vi "Remote Systems Demo.vi"() -> ()   [LabVIEW 2020]
uses:
  Dynamic Combobox/Dynamic Combobox/Options.ctl
  Remote Systems.lvclass
  C:/dev/NI/Dynamic Combobox/Dynamic Combobox/Dynamic Values/Dynamic Values.lvclass
  Dynamic Combobox/Dynamic Combobox/Dynamic Combobox.lvclass
  <vilib>/nisyscfg/nisyscfg.lvlib
  <resource>/objmgr/nisysapi.rc
panel:
  out "Serial Number":string
  out "Product Name":string
  out "Product ID":i32 format="%.0x"
  out "Firmware Revision":string
  out "Device Class":string
  out "error out":errorcluster
  in  "Cancel Button":bool
  in  "OK Button":bool
  in  "System Selection":string(combo)
  out "Selected System":string
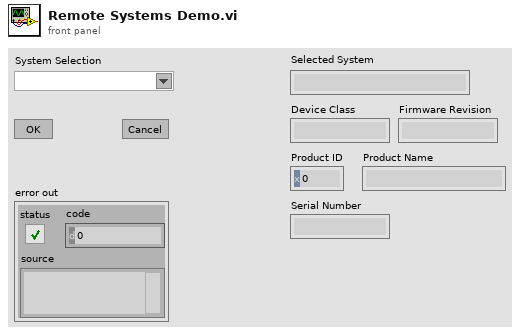
[diagram p1: front panel]
types:
  T1 = typedef "Dynamic Combobox.lvlib/Dynamic Combobox.lvclass/Options.ctl" = cluster{"Browse Entry":bool, "Refresh Entry":bool}
  T2 = typedef "Dynamic Combobox.lvlib/Dynamic Combobox.lvclass/Dynamic Combobox Events.ctl" = cluster{"Selection":refnum<user-event>, "Error":refnum<user-event>}
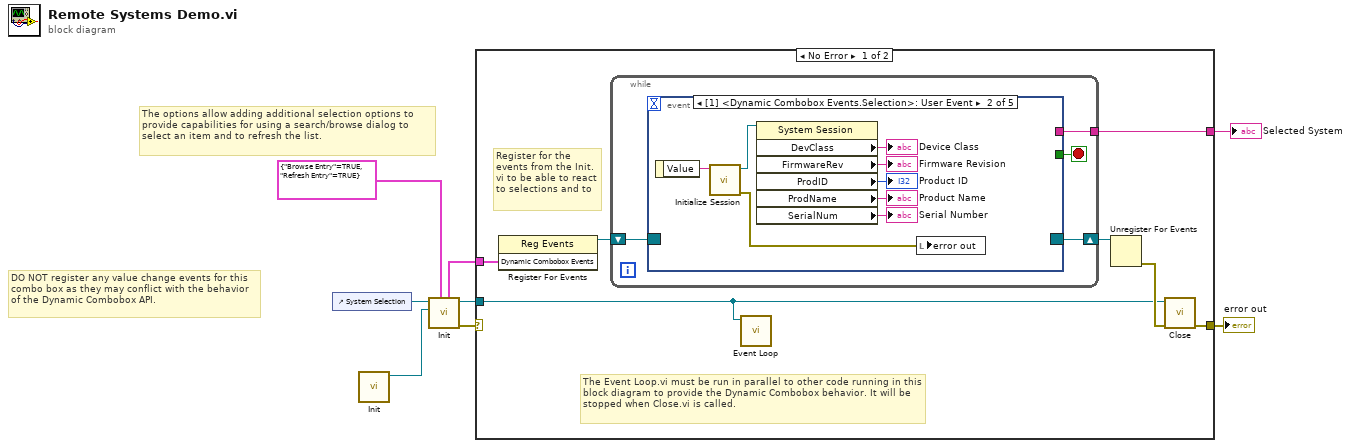
[diagram p0: block diagram]
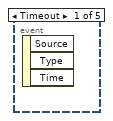
[diagram p2: hidden frame]
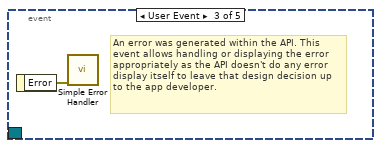
[diagram p3: hidden frame]
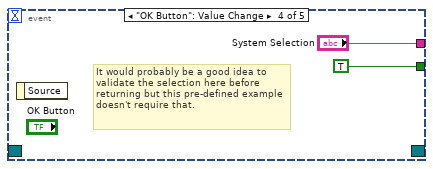
[diagram p4: hidden frame]
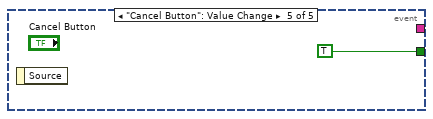
[diagram p5: hidden frame]
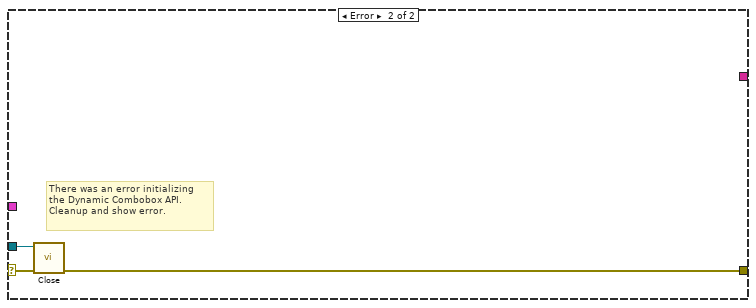
[diagram p6: hidden frame]
diagram:
  # "DO NOT register any value change events for this combo box as they may conflict with the behavior of the Dynamic Combobox API."
  # "The options allow adding additional selection options to provide capabilities for using a search/browse dialog to select an item and to refresh the list."
  n1 = control-ref of="System Selection"() -> (w8:refnum<vi>)
  n2 = call "Init.vi"() -> ("Remote Systems out"=w2:refnum<class "Remote Systems.lvclass">)  [unwired: 10 in, 1 out]
  n3 = call "Init.vi"("Options (None)"=T1 {"Browse Entry"=TRUE, "Refresh Entry"=TRUE} ("Options (Refresh First Open)"), "Dynamic Values"=w2, "Combobox"=w8) -> ("error out"=w3:errorcluster, "Dynamic Combobox out"=w4:refnum<class "Dynamic Combobox.lvclass">, "Dynamic Combobox Events"=w7:T2)  [unwired: 6 in]
  n4 = case shown="No Error" w3 {
    selector: w3 -> [_ w33]
    tunnel: w7 -> [w15 _]
    tunnel: [w12 _] -> w5
    tunnel: w4 -> [w9 w34]
    tunnel: [w11 w32] -> w1
    frame No Error {
      # "The Event Loop.vi must be run in parallel to other code running in this block diagram to provide the Dynamic Combobox behavior. It will be stopped when Close.vi is called."
      # "Register for the events from the Init.vi to be able to react to selections and to"
      n5 = register-events(w15) -> (reference out=w14:refnum<event-registration>)  [unwired: 2 in, 1 out]
      n6 = while {
        shift-right: [w18] -> w13
        shift-left: w14 -> [w19]
        tunnel: [w16] -> w12
        stop <- w17 stop-if-true
        n7 = event shown="[1] <Dynamic Combobox Events.Selection>: User Event" {
          selector: w19 -> [_ _ _ _ _]
          dyn-events: [_ _ _ _ _] -> w18
          timeout: _ -> [_ _ _ _ _]
          tunnel: [_ _ _ TRUE ("Valid") TRUE ("Valid")] -> w17
          tunnel: [_ _ _ "System Selection" _] -> w16
          event Timeout {
            n8 = event-data() -> ()  [unwired: 1 in, 3 out]
          }
          event User Event {
            n9 = event-data() -> ("Value"=w27:string)  [unwired: 1 in]
            n10 = call <vilib>:"Initialize Session.vi"("Target (localhost)"=w27) -> ("error out"=w26:errorcluster, "Session out"=w25:refnum<k21>)  [unwired: 9 in]
            n11 = property class="System Session"(reference=w25) -> ("DevClass"=→"Device Class":string, "FirmwareRev"=→"Firmware Revision":string, "ProdID"=→"Product ID":i32, "ProdName"=→"Product Name":string, "SerialNum"=→"Serial Number":string)  [unwired: 1 in, 2 out]
            n12 = local write "error out"(w26) -> ()
          }
          event User Event {
            # "An error was generated within the API. This event allows handling or displaying the error appropriately as the API doesn't do any error display itself to leave that design decision up to the app developer."
            n13 = event-data() -> ("Error"=w28:errorcluster)  [unwired: 1 in]
            n14 = call <vilib>:"Simple Error Handler.vi"("error in (no error)"=w28) -> ()  [unwired: 4 in, 5 out]
          }
          event "OK Button": Value Change {
            # "It would probably be a good idea to validate the selection here before returning but this pre-defined example doesn't require that."
            n15 = event-data() -> ()  [unwired: 1 in, 1 out]
          }
          event "Cancel Button": Value Change {
            n16 = event-data() -> ()  [unwired: 1 in, 1 out]
          }
        }
      }
      n17 = call "Event Loop.vi"("Dynamic Combobox in"=w9) -> ()  [unwired: 10 in, 1 out]
      n18 = Unregister For Events(event registration refnum=w13) -> (error out=w10:errorcluster)  [unwired: 1 in]
      n19 = call "Close.vi"("error in (no error)"=w10, "Dynamic Combobox in"=w9) -> ("error out"=w11:errorcluster)  [unwired: 9 in]
    }
    frame Error {
      # "There was an error initializing the Dynamic Combobox API. Cleanup and show error."
      n20 = call "Close.vi"("error in (no error)"=w33, "Dynamic Combobox in"=w34) -> ("error out"=w32:errorcluster)  [unwired: 9 in]
    }
  }
  "Selected System" <- w5
  "error out" <- w1
